vi "Pre-Process Transparency.vi"() -> ()   [LabVIEW 2018]
doc: "Demonstrates how to overlay a image with a transparent image\n\nLabVIEW only recognizes binary states for pixels: full transparency or full opaqueness\nKB 3T9924OA: Reading 32-Bit PNG Files with LabVIEW\nhttp://digital.ni.com/public.nsf/allkb/EEDD9D6EAB559B73862570F200584773?OpenDocument"
panel:
  out "Mask":T1(plugin-control)
  out "Processed":T1(plugin-control)
  out "Origin":picture
  in  "path to PNG file":path
  # "Overview: Demonstrates how to overlay a image with a transparent image\nRequirements: LabVIEW 2012 Base Development System (or compatible)\n                             Vision Development Module 2012 (or compatible)\nInstructions: \n1. Select whether the transparency of the overlay image shall be preserved\n2. Run the VI"
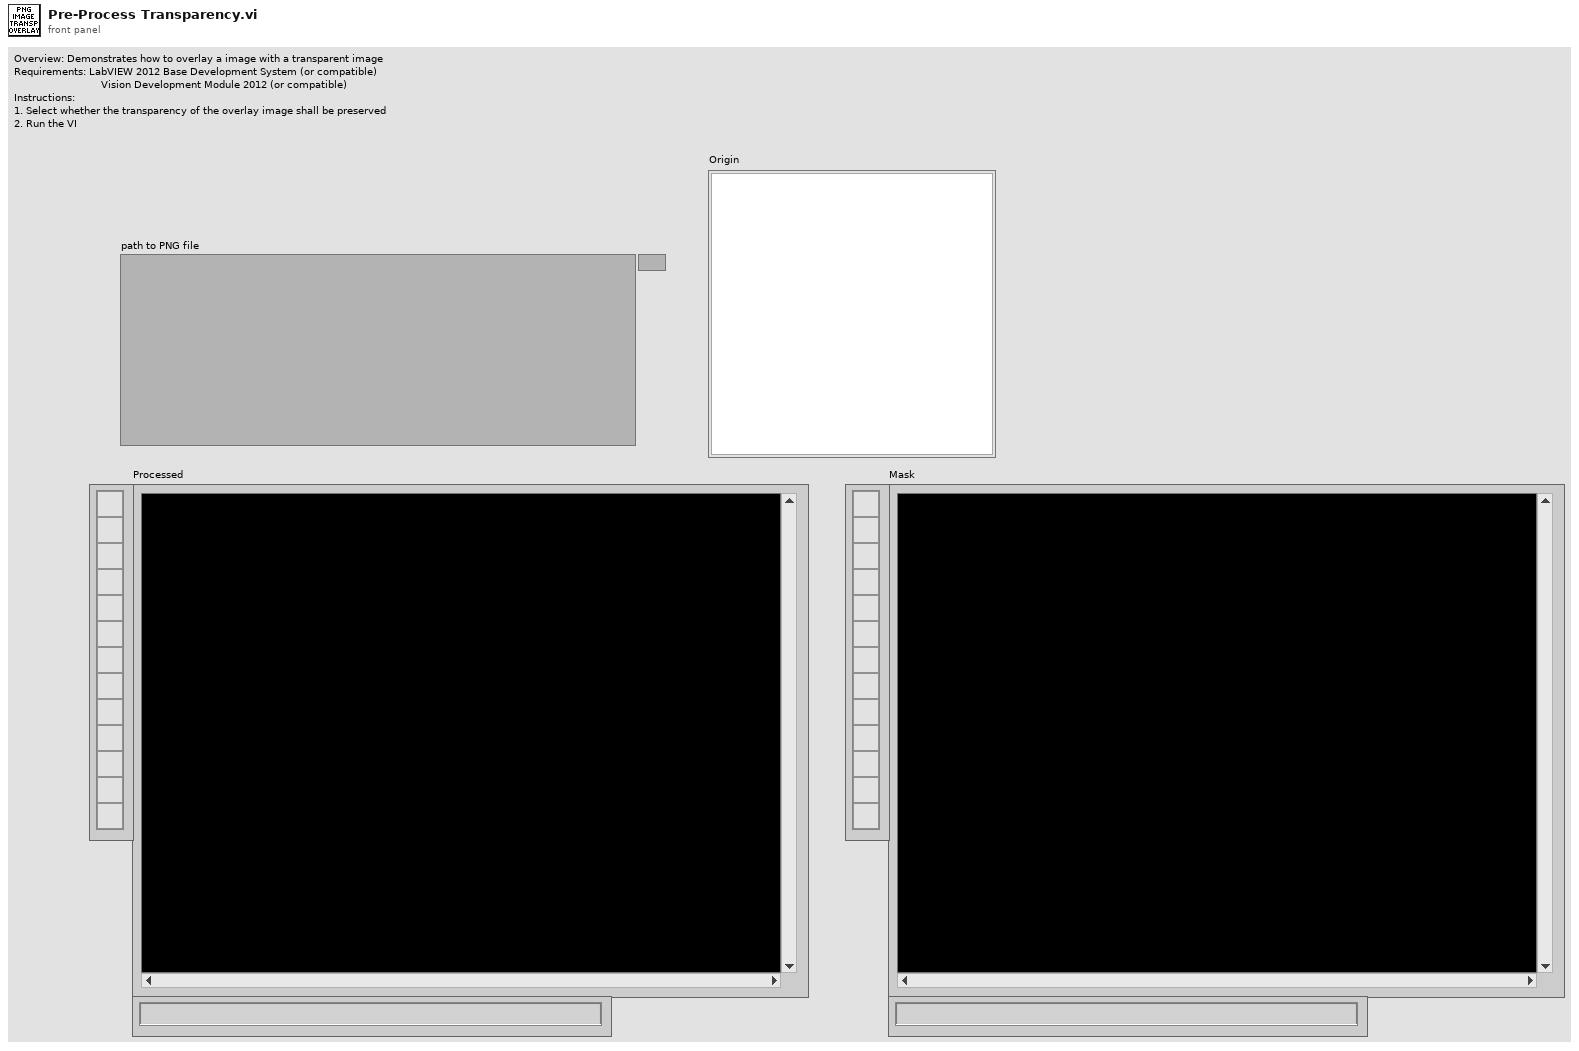
[diagram p1: front panel]
types:
  T1 = typedef "IMAQ Image.ctl" = refnum<image>
  T2 = typedef "imagedata.ctl" = cluster{"image type":i32, "image depth":i32, "image":u8[], "mask":u8[], "colors":u32[], "Rectangle":cluster{"left":i16, "top":i16, "right":i16, "bottom":i16}}
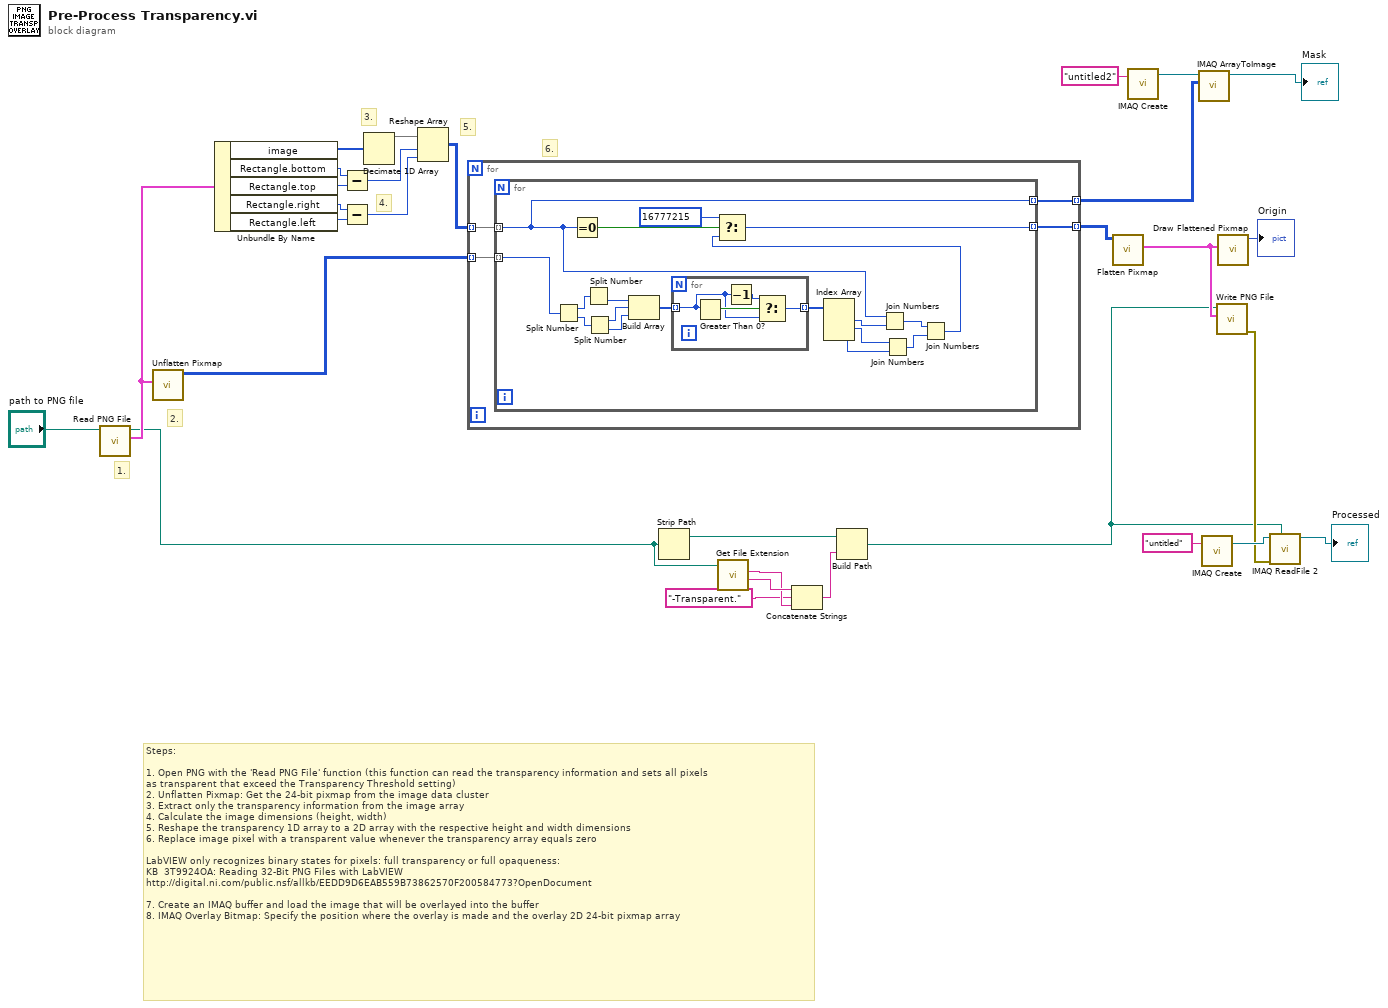
[diagram p0: block diagram]
diagram:
  # "6."
  # "5."
  # "4."
  # "3."
  # "2."
  # "1."
  # "Steps:\n\n1. Open PNG with the 'Read PNG File' function (this function can read the transparency information and sets all pixels\nas transparent that exceed the Transparency Threshold setting)\n2. Unflatten Pixmap: Get the 24-bit pixmap from the image data cluster\n3. Extract only the transparency information from the image array\n4. Calculate the image dimensions (height, width)\n5. Reshape the transparency 1D array to a 2D array with the respective height and width dimensions\n6. Replace image pixel with a transparent value whenever the transparency array equals zero\n\nLabVIEW only recognizes binary states for pixels: full transparency or full opaqueness:\nKB  3T9924OA: Reading 32-Bit PNG Files with LabVIEW\nhttp://digital.ni.com/public.nsf/allkb/EEDD9D6EAB559B73862570F200584773?OpenDocument\n\n7. Create an IMAQ buffer and load the image that will be overlayed into the buffer\n8. IMAQ Overlay Bitmap: Specify the position where the overlay is made and the overlay 2D 24-bit pixmap array"
  n1 = call <vilib>:"Read PNG File.vi"("path to PNG file"="path to PNG file") -> ("image data"=w30:T2, "path"=w1:path)  [unwired: 8 in, 1 out]
  n2 = call <vilib>:"Unflatten Pixmap.vi"("image data"=w30) -> ("24-bit pixmap"=w29:u32[][])  [unwired: 4 in, 6 out]
  n3 = Unbundle By Name(w30) -> ("image"=w28:u8[], "Rectangle.bottom"=w25:i16, "Rectangle.top"=w24:i16, "Rectangle.right"=w22:i16, "Rectangle.left"=w23:i16)
  n4 = Subtract(x=w25, y=w24) -> (x-y=w21:i16)
  n5 = Subtract(x=w22, y=w23) -> (x-y=w20:i16)
  n6 = Decimate 1D Array(w28) -> (w27:u8[])  [unwired: 3 out]
  n7 = Reshape Array(w27, w21, w20) -> (w26:u8[][])
  n8 = for {
    tunnel: [w34] -> w19 mode=indexing
    tunnel: w26 -> [w33] mode=indexing
    tunnel: w29 -> [w32] mode=indexing
    tunnel: [w31] -> w10 mode=indexing
    n9 = for {
      tunnel: [w51] -> w34 mode=indexing
      tunnel: w33 -> [w36] mode=indexing
      tunnel: w32 -> [w50] mode=indexing
      tunnel: [w36] -> w31 mode=indexing
      n10 = Split Number(x=w50) -> (hi(x)=w48:u16, lo(x)=w49:u16)
      n11 = Equal To 0?(x=w36) -> (x = 0?=w52:bool)
      n12 = Split Number(x=w48) -> (lo(x)=w47:u8)  [unwired: 1 out]
      n13 = Split Number(x=w49) -> (hi(x)=w46:u8, lo(x)=w45:u8)
      n14 = Build Array(w47, w46, w45) -> (w44:u8[])
      n15 = for {
        tunnel: w44 -> [w54] mode=indexing
        tunnel: [w53] -> w43 mode=indexing
        n16 = Greater Than 0?(x=w54) -> (x > 0?=w56:bool)
        n17 = Decrement(x=w54) -> (x-1=w55:u8)
        n18 = Select(t=w55, s=w56, f=w54) -> (s? t:f=w53:u8)
      }
      n19 = Index Array(array=w43) -> (element #1=w41:u8, element #2=w40:u8, element #3=w39:u8)  [unwired: 3 in]
      n20 = Join Numbers(hi=w36, lo=w41) -> ((hi.lo)=w37:u16)
      n21 = Join Numbers(hi=w40, lo=w39) -> ((hi.lo)=w38:u16)
      n22 = Join Numbers(hi=w37, lo=w38) -> ((hi.lo)=w42:u32)
      n23 = Select(t=u32 16777215, s=w52, f=w42) -> (s? t:f=w51:u32)
    }
  }
  n24 = Strip Path(path=w1) -> (stripped path=w7:path)  [unwired: 1 out]
  n25 = call <vilib>:"Get File Extension.vi"("file"=w1) -> ("filename without extension"=w6:string, "lowercase file extension"=w5:string)  [unwired: 6 in, 3 out]
  n26 = Concatenate Strings(w6, "-Transparent." ("string"), w5) -> (w3:string)
  n27 = Build Path(base path=w7, name or relative path=w3) -> (appended path=w2:path)
  n28 = call <vilib>:"Flatten Pixmap.vi"("24-bit pixmap"=w19) -> ("image data"=w17:T2)  [unwired: 10 in]
  n29 = call "IMAQ Create"("Image Name"="untitled2") -> ("New Image"=w11:T1)  [unwired: 4 in, 1 out]
  n30 = call "IMAQ ArrayToImage"("Image Pixels (U8)"=w10, "Image"=w11) -> ("Image Out"=→"Mask":T1)  [unwired: 8 in, 1 out]
  n31 = call "IMAQ Create"("Image Name"="untitled") -> ("New Image"=w15:T1)  [unwired: 4 in, 1 out]
  n32 = call <vilib>:"Write PNG File.vi"("image data"=w17, "path to PNG file"=w2) -> ("error out"=w14:errorcluster)  [unwired: 8 in, 1 out]
  n33 = call <vilib>:"Draw Flattened Pixmap.vi"("image data"=w17) -> ("new picture"=→"Origin":picture)  [unwired: 8 in]
  n34 = call "IMAQ ReadFile 2"("File Path"=w2, "error in (no error)"=w14, "Image"=w15) -> ("Image Out"=→"Processed":T1)  [unwired: 4 in, 4 out]
